vi "总磷氨氮插入数据.vi"(0 "table":string, 1 "关键参数":T1, 5 "data":T3={"时间标识"=timestamp(0 s since 1904-01-01), "测量模式"=enum."水样测试", "数据标记表"="N", "监测值"=0.0, "单位"=0, "数据标识"="", "因子编码"=0, "标样参考值"=0.0, "F0"=0.0, "F1"=0.0, "F2"=0.0, "F3"=0.0, "F4"=0.0, "F5"=0.0, "F6"=0.0, "F7"=0.0, "X"=0.0, "温度"=0.0, "湿度"=0.0, "量程标识"="", "SN"="", "跨度值"=0.0} {"单位" items=["μg/L", "mg/L", "ppm", "mg/m3", "cm", "ppb", "μg/m3", "%", "nmol/mol", "μmol/mol", "MPN/L", "MPN/100ml", "ng/m3", "NTU", "无量纲", "ms/cm", "μs/cm"]}, 11 "error in (no error)":errorcluster) -> (15 "error out":errorcluster)   [LabVIEW 2016, in "斯坦道氨氮.lvlib"]
uses:
  <vilib>/Utility/sysdir.llb/System Directory Type.ctl
  <vilib>/Utility/error.llb/DialogType.ctl
  <vilib>/addons/database/Auxilliary.llb/DB Tools Column Info.ctl
  <vilib>/addons/database/Auxilliary.llb/DB Tools DataTypes.ctl
  <vilib>/addons/database/Connection.llb/DB Tools Open Connec (String).vi
  <vilib>/addons/database/Connection.llb/Conn Execute.vi
  <vilib>/addons/database/Recordset.llb/Rec Fetch Recordset Data (R).vi
  <vilib>/addons/database/Recordset.llb/Rec Destroy - Connection.vi
  <vilib>/addons/database/NI_Database_API.lvlib
  <vilib>/Utility/VariantDataType/VariantType.lvlib
panel:
  out "data输出":T2
  out "为空？":bool
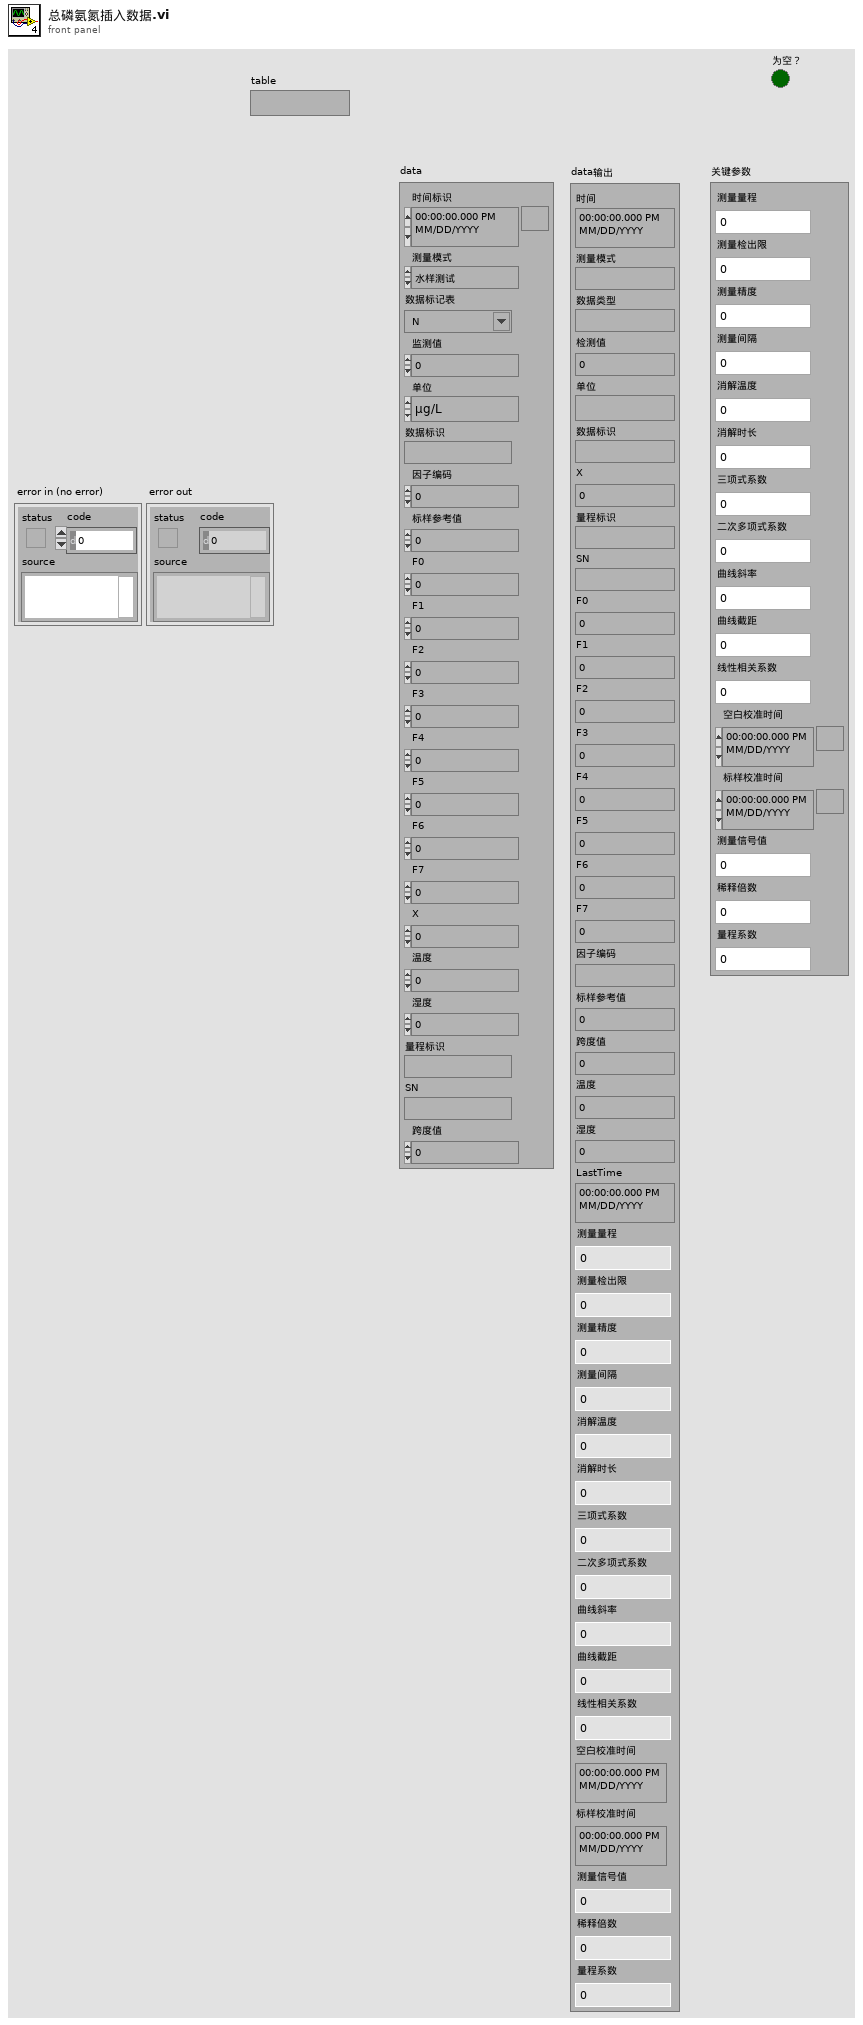
[diagram p1: front panel]
types:
  T1 = typedef "斯坦道氨氮.lvlib/关键参数.ctl" = cluster{"测量量程":sgl, "测量检出限":sgl, "测量精度":sgl, "测量间隔":sgl, "消解温度":sgl, "消解时长":sgl, "三项式系数":sgl, "二次多项式系数":sgl, "曲线斜率":sgl, "曲线截距":sgl, "线性相关系数":sgl, "空白校准时间":timestamp, "标样校准时间":timestamp, "测量信号值":sgl, "稀释倍数":sgl, "量程系数":sgl}
  T2 = cluster{"时间":timestamp, "测量模式":string, "数据类型":string, "检测值":sgl, "单位":string, "数据标识":string, "X":sgl, "量程标识":string, "SN":string, "F0":sgl, "F1":sgl, "F2":sgl, "F3":sgl, "F4":sgl, "F5":sgl, "F6":sgl, "F7":sgl, "因子编码":string, "标样参考值":sgl, "跨度值":sgl, "温度":sgl, "湿度":sgl, "LastTime":timestamp, "测量量程":sgl, "测量检出限":sgl, "测量精度":sgl, "测量间隔":sgl, "消解温度":sgl, "消解时长":sgl, "三项式系数":sgl, "二次多项式系数":sgl, "曲线斜率":sgl, "曲线截距":sgl, "线性相关系数":sgl, "空白校准时间":timestamp, "标样校准时间":timestamp, "测量信号值":sgl, "稀释倍数":sgl, "量程系数":sgl}
  T3 = cluster{"时间标识":timestamp, "测量模式":enum16{"维护数据", "水样测试", "标样核查", "零点核查", "跨度核查", "空白测试", "平行样测试", "加标回收", "空白校准", "标样校准", "初始化（清洗）"}, "数据标记表":string, "监测值":sgl, "单位":u16, "数据标识":string, "因子编码":u32, "标样参考值":sgl, "F0":sgl, "F1":sgl, "F2":sgl, "F3":sgl, "F4":sgl, "F5":sgl, "F6":sgl, "F7":sgl, "X":sgl, "温度":sgl, "湿度":sgl, "量程标识":string, "SN":string, "跨度值":sgl}
  T4 = typedef "DialogType.ctl" = u16
  T5 = typedef "System Directory Type.ctl" = i32
  T6 = typedef "NI_Database_API.lvlib/Conn ObjectReference.ctl" = refnum<k1>
  T7 = typedef "NI_Database_API.lvlib/Rec ObjectReference.ctl" = refnum<k1>
  T8 = typedef "NI_Database_API.lvlib/DB Tools Column Info.ctl" = cluster{"column name":string, "data type":T9, "size":i32, "allow null?":bool}
  T9 = typedef "NI_Database_API.lvlib/DB Tools DataTypes.ctl" = enum16{"String", "Long (I32)", "Single (SGL)", "Double (DBL)", "Date/Time", "Binary"}
  T10 = enum16{"维护数据", "水样测试", "标样核查", "零点核查", "跨度核查", "空白测试", "平行样测试", "加标回收", "空白校准", "标样校准", "初始化（清洗）"}
  T11 = cluster{"测量量程":dbl, "测量精度":dbl, "测量间隔":dbl, "消解温度":dbl, "消解时长":dbl, "空白校准时间":timestamp, "曲线截距":dbl, "曲线斜率":dbl, "测量检出限":dbl, "测量信号值":dbl, "线性相关系数":dbl, "二次多项式系数":dbl, "标样校准时间":timestamp, "稀释倍数":dbl, "三项式系数":dbl, "空白标定系数":dbl, "量程系数":dbl, "F0/ORPA":dbl, "F1/ORPB":dbl, "F2/ORPK":dbl, "F3":dbl, "F4":dbl, "F5":dbl, "F6":dbl, "F7":dbl, "X0/滴定数":dbl, "量程":dbl}
  T12 = typedef "VariantType.lvlib/Type.ctl" = enum8{"Invalid Type", "Void", "I8", "I16", "I32", "I64", "U8", "U16", "U32", "U64", "Single Float", "Double Float", "Extended Float", "Single Complex", "Double Complex", "Extended Complex", "Enum U8", "Enum U16", "Enum U32", "Enum U64", "Single Float With Unit", "Double Float With Unit", "Extended Float With Unit", "Single Complex with Unit", "Double Complex with Unit", "Extended Complex with Unit", "Boolean", "String", "Path", "Picture", "Tag", "Array", "Cluster", "Variant", "LV Variant", "Waveform", "Timestamp", "Digital Waveform", "Digital Data", "ExpressData", "Refnum", "External Data", "VI", "Poly VI", "LabVIEW Class Instance", "Fixed Point"}
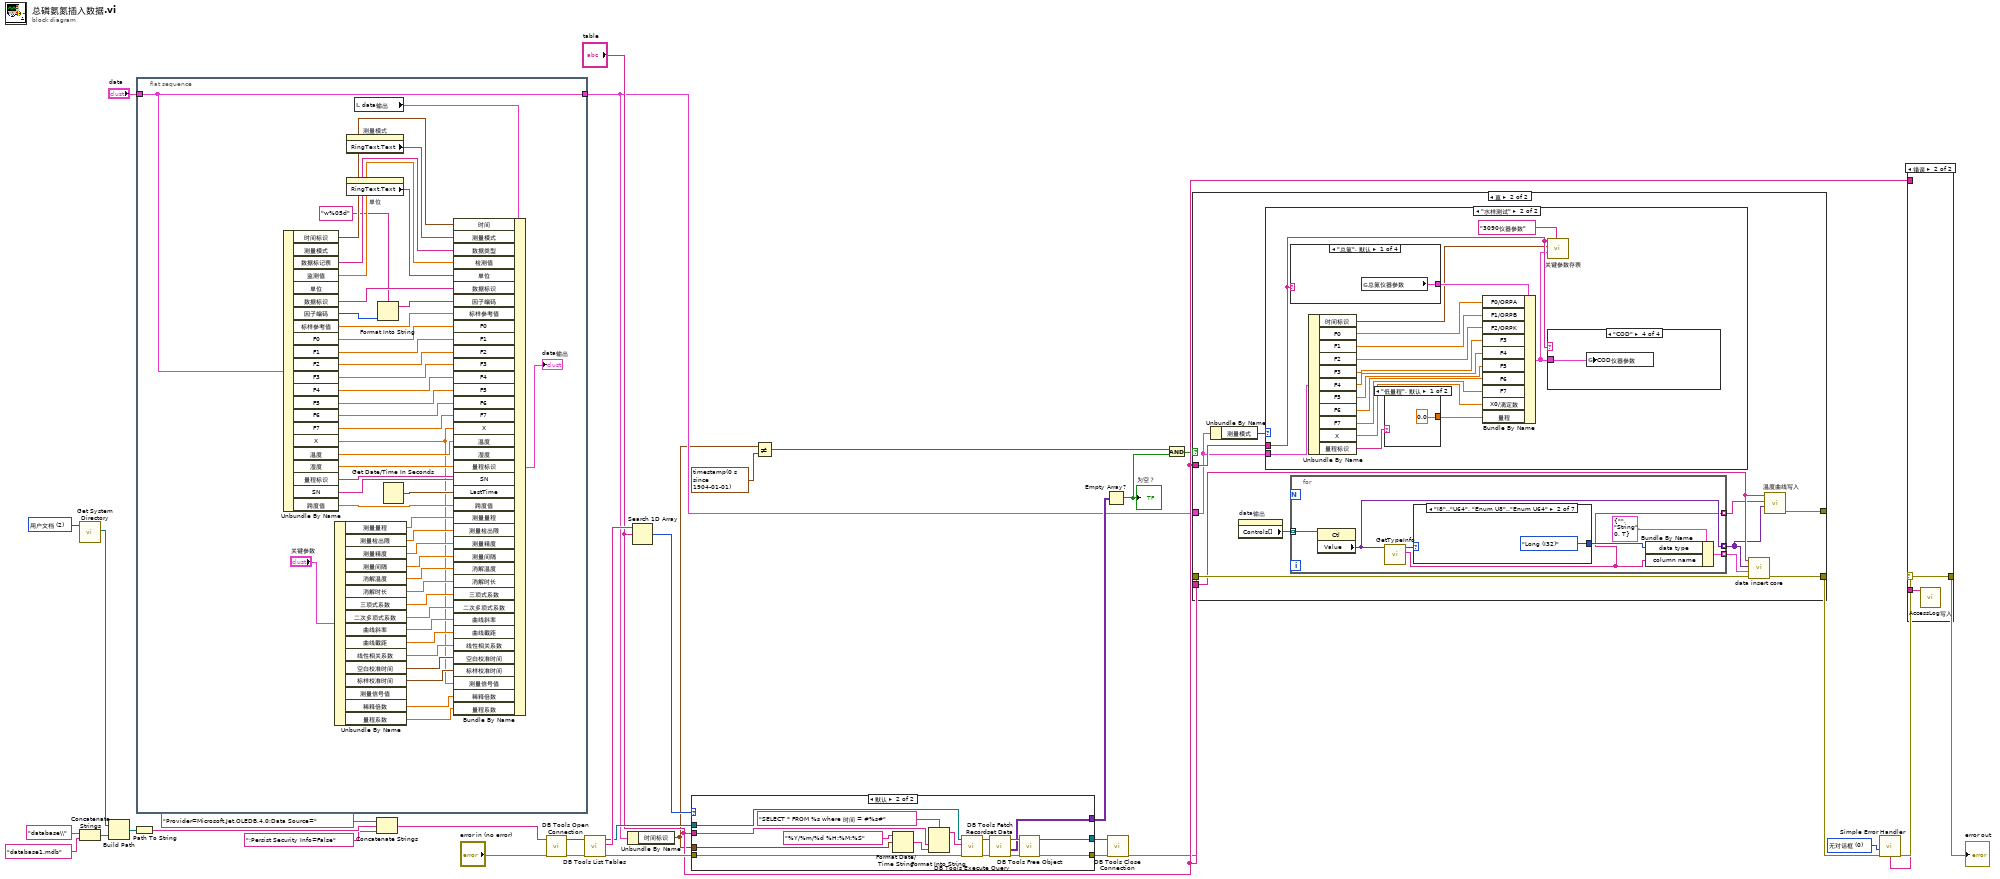
[diagram p0: block diagram]
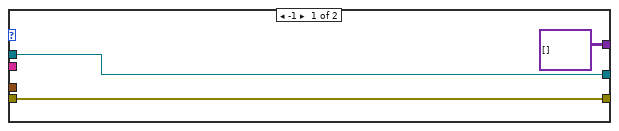
[diagram p3: hidden frame]
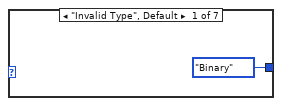
[diagram p5: hidden frame]
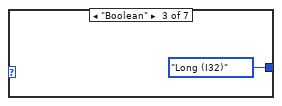
[diagram p6: hidden frame]
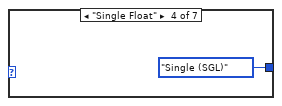
[diagram p7: hidden frame]
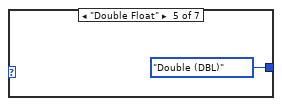
[diagram p8: hidden frame]
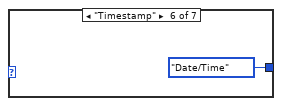
[diagram p9: hidden frame]
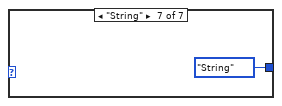
[diagram p10: hidden frame]
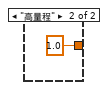
[diagram p12: hidden frame]
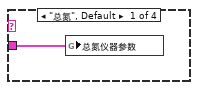
[diagram p13: hidden frame]
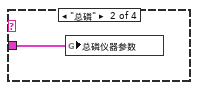
[diagram p14: hidden frame]
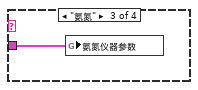
[diagram p15: hidden frame]
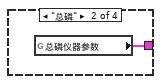
[diagram p16: hidden frame]
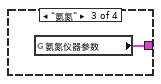
[diagram p17: hidden frame]
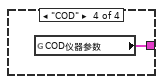
[diagram p18: hidden frame]
diagram:
  w15 = T4 0 items=["无对话框", "确定信息", "继续或停止信息", "确定信息＋警告", "继续/停止+警告"] ("type of dialog (OK msg:1)")
  w33 = T5 2 items=["用户目录"=0, "用户桌面"=1, "用户文档"=2, "用户应用程序数据"=3, "用户设置"=4, "用户临时目录"=5, "公共文档"=6, "公共应用程序数据"=7, "公共设置"=8, "公共缓存"=13, "系统核心库"=9, "系统安装库"=10, "应用程序文件"=11, "启动盘根目录"=12] ("system directory type")
  n1 = call <vilib>:"Get System Directory.vi"("system directory type"=w33) -> ("system directory"=w31:path)  [unwired: 10 in]
  n2 = Concatenate Strings("database\\" ("condition"), "database1.mdb" ("database")) -> (w25:string)
  n3 = Build Path(base path=w31, name or relative path=w25) -> (appended path=w30:path)
  n4 = Path To String(path=w30) -> (string=w29:string)
  n5 = flat-sequence {
    tunnel: "data" -> [w57]
    tunnel: [w57] -> w9
    frame #0 {
      n6 = Unbundle By Name(w57) -> ("时间标识"=w77:timestamp, "数据标记表"=w75:string, "监测值"=w74:sgl, "数据标识"=w72:string, "因子编码"=w56:u32, "标样参考值"=w71:sgl, "F0"=w70:sgl, "F1"=w69:sgl, "F2"=w68:sgl, "F3"=w67:sgl, "F4"=w66:sgl, "F5"=w65:sgl, "F6"=w64:sgl, "F7"=w63:sgl, "X"=w35:sgl, "温度"=w62:sgl, "湿度"=w61:sgl, "量程标识"=w60:string, "SN"=w59:string, "跨度值"=w52:sgl)  [unwired: 2 out]
      n7 = Unbundle By Name("关键参数") -> ("测量量程"=w50:sgl, "测量检出限"=w49:sgl, "测量精度"=w48:sgl, "测量间隔"=w47:sgl, "消解温度"=w46:sgl, "消解时长"=w45:sgl, "三项式系数"=w44:sgl, "二次多项式系数"=w43:sgl, "曲线斜率"=w42:sgl, "曲线截距"=w41:sgl, "线性相关系数"=w40:sgl, "空白校准时间"=w39:timestamp, "标样校准时间"=w38:timestamp, "稀释倍数"=w37:sgl, "量程系数"=w36:sgl)  [unwired: 1 out]
      n8 = property on="测量模式" class="Enum (严格)"() -> ("RingText.Text"=w76:string)  [unwired: 2 in, 2 out]
      n9 = property on="单位" class="Ring (严格)"() -> ("RingText.Text"=w73:string)  [unwired: 2 in, 2 out]
      n10 = local read "data输出"() -> (w53:T2)
      n11 = Format Into String(format string="w%05d" ("格式字符串"), w56) -> (resulting string=w54:string)  [unwired: 2 in, 1 out]
      n12 = Get Date/Time In Seconds() -> (seconds since 1Jan1904=w58:timestamp)
      n13 = Bundle By Name(cluster=w53, "时间"=w77, "测量模式"=w76, "数据类型"=w75, "检测值"=w74, "单位"=w73, "数据标识"=w72, "因子编码"=w54, "标样参考值"=w71, "F0"=w70, "F1"=w69, "F2"=w68, "F3"=w67, "F4"=w66, "F5"=w65, "F6"=w64, "F7"=w63, "X"=w35, "温度"=w62, "湿度"=w61, "量程标识"=w60, "SN"=w59, "LastTime"=w58, "跨度值"=w52, "测量量程"=w50, "测量检出限"=w49, "测量精度"=w48, "测量间隔"=w47, "消解温度"=w46, "消解时长"=w45, "三项式系数"=w44, "二次多项式系数"=w43, "曲线斜率"=w42, "曲线截距"=w41, "线性相关系数"=w40, "空白校准时间"=w39, "标样校准时间"=w38, "测量信号值"=w35, "稀释倍数"=w37, "量程系数"=w36) -> (→"data输出":T2)
    }
  }
  n14 = Concatenate Strings("Provider=Microsoft.Jet.OLEDB.4.0;Data Source=" ("condition"), w29, ";Persist Security Info=False" ("condition")) -> (w27:string)
  n15 = call-poly <vilib>:"DB Tools Open Connection.vi"("error in (no error)"="error in (no error)", "connection information"=w27) -> ("error out"=w23:errorcluster, "connection reference"=w24:T6)  [unwired: 6 in]
  n16 = call <vilib>:"DB Tools List Tables.vi"("error in (no error)"=w23, "connection reference"=w24) -> ("error out"=w17:errorcluster, "tables"=w22:string[], "connection reference out"=w18:T6)  [unwired: 3 in]
  n17 = Unbundle By Name(w9) -> ("时间标识"=w7:timestamp)
  n18 = Search 1D Array(1D array=w22, element="table") -> (index of element=w19:i32)  [unwired: 1 in]
  n19 = case shown="默认" w19 {
    tunnel: [variant[][] [] ("recordset data") w92] -> w16
    tunnel: [w81 w83] -> w4
    tunnel: [w80 w91] -> w3
    tunnel: w18 -> [w81 w87]
    tunnel: w17 -> [w80 w86]
    tunnel: "table" -> [_ w85]
    tunnel: w7 -> [_ w82]
    frame -1 {
    }
    frame Default {
      n20 = Format Date/Time String(time format string (%c)="%Y/%m/%d %H:%M:%S" ("时间格式字符串(%c)"), seconds (now)=w82) -> (date/time string=w88:string)  [unwired: 1 in]
      n21 = Format Into String(format string="SELECT * FROM %s where 时间 = #%s#" ("格式字符串"), w85, w88) -> (resulting string=w90:string)  [unwired: 2 in, 1 out]
      n22 = call-poly <vilib>:"DB Tools Execute Query.vi"("error in (no error)"=w86, "SQL query"=w90, "connection reference"=w87) -> ("error out"=w93:errorcluster, "recordset reference"=w96:T7)  [unwired: 5 in]
      n23 = call-poly <vilib>:"DB Tools Fetch Recordset Data.vi"("error in (no error)"=w93, "recordset reference"=w96) -> ("error out"=w94:errorcluster, "recordset data"=w92:variant[][], "recordset reference out"=w95:T7)  [unwired: 3 in]
      n24 = call-poly <vilib>:"DB Tools Free Object.vi"("error in (no error)"=w94, "recordset reference"=w95) -> ("error out"=w91:errorcluster, "connection reference"=w83:T6)  [unwired: 8 in]
    }
  }
  n25 = Not Equal?(x=w7, y=timestamp(0 s since 1904-01-01)) -> (x != y?=w5:bool)
  n26 = Empty Array?(array=w16) -> (empty?=w20:bool)
  "为空？" <- w20
  n27 = call <vilib>:"DB Tools Close Connection.vi"("error in (no error)"=w3, "connection reference"=w4) -> ("error out"=w2:errorcluster)  [unwired: 5 in]
  n28 = And(x=w5, y=w20) -> (x .and. y?=w6:bool)
  n29 = case shown="真" w6 {
    tunnel: "table" -> [_ w101]
    tunnel: w9 -> [_ w106]
    tunnel: w2 -> [w97 w102]
    tunnel: [w97 w107] -> w1
    tunnel: "table" -> [_ w108]
    tunnel: [_ w100] -> _
    frame False {
    }
    frame True {
      n30 = Unbundle By Name(w106) -> ("测量模式"=w105:T10)
      n31 = property on="data输出" class="Clust (严格)"() -> ("Controls[]"=w104:refnum<vi>[])  [unwired: 2 in, 2 out]
      n32 = case shown="\"水样测试\"" w105 {
        tunnel: w106 -> [_ w138]
        tunnel: w108 -> [_ w136]
        frame "维护数据", Default {
        }
        frame "水样测试" {
          n33 = case shown="\"总氮\", 默认" w136 {
            tunnel: [w146 w147 w148 w149] -> w137
            frame "总氮", Default {
              n34 = global read "总磷总氮断电保存全局变量.vi" "总氮仪器参数"() -> (w146:T11)
            }
            frame "总磷" {
              n35 = global read "总磷总氮断电保存全局变量.vi" "总磷仪器参数"() -> (w147:T11)
            }
            frame "氨氮" {
              n36 = global read "总磷总氮断电保存全局变量.vi" "氨氮仪器参数"() -> (w148:T11)
            }
            frame "COD" {
              n37 = global read "总磷总氮断电保存全局变量.vi" "COD仪器参数"() -> (w149:T11)
            }
          }
          n38 = Unbundle By Name(w138) -> ("时间标识"=w134:timestamp, "F0"=w123:sgl, "F1"=w124:sgl, "F2"=w125:sgl, "F3"=w126:sgl, "F4"=w127:sgl, "F5"=w128:sgl, "F6"=w129:sgl, "F7"=w130:sgl, "X"=w131:sgl, "量程标识"=w133:string)
          n39 = case shown="\"低量程\", 默认" w133 {
            tunnel: [0.0 1.0] -> w132
            frame "低量程", Default {
            }
            frame "高量程" {
            }
          }
          n40 = Bundle By Name(cluster=w137, "F0/ORPA"=w123, "F1/ORPB"=w124, "F2/ORPK"=w125, "F3"=w126, "F4"=w127, "F5"=w128, "F6"=w129, "F7"=w130, "X0/滴定数"=w131, "量程"=w132) -> (w135:T11)
          n41 = call "关键参数存表.vi"("table"="3090仪器参数", "仪器参数"=w135, "datatime"=w134, "仪器名称"=w136) -> ()  [unwired: 7 in, 1 out]
          n42 = case shown="\"COD\"" w136 {
            tunnel: w135 -> [w142 w143 w144 w145]
            frame "总氮", Default {
              n43 = global write "总磷总氮断电保存全局变量.vi" "总氮仪器参数"(w142) -> ()
            }
            frame "总磷" {
              n44 = global write "总磷总氮断电保存全局变量.vi" "总磷仪器参数"(w143) -> ()
            }
            frame "氨氮" {
              n45 = global write "总磷总氮断电保存全局变量.vi" "氨氮仪器参数"(w144) -> ()
            }
            frame "COD" {
              n46 = global write "总磷总氮断电保存全局变量.vi" "COD仪器参数"(w145) -> ()
            }
          }
        }
      }
      n47 = for {
        tunnel: w104 -> [w115] mode=indexing
        tunnel: [w110] -> w98 mode=indexing
        tunnel: [w111] -> w103 mode=indexing
        tunnel: [w109] -> w99 mode=indexing
        n48 = property class="Ctl"(reference=w115) -> ("Value"=w110:variant)  [unwired: 1 in, 2 out]
        n49 = call <vilib>:"GetTypeInfo.vi"("Variant"=w110) -> ("Name"=w109:string, "Type Enum"=w113:T12)  [unwired: 6 in, 3 out]
        n50 = case shown="\"I8\"..\"U64\", \"Enum U8\"..\"Enum U64\"" w113 {
          tunnel: [DB_Tools_DataTypes."Binary" ("data type") DB_Tools_DataTypes."Long (I32)" ("data type") DB_Tools_DataTypes."Long (I32)" ("data type") DB_Tools_DataTypes."Single (SGL)" ("data type") DB_Tools_DataTypes."Double (DBL)" ("data type") DB_Tools_DataTypes."Date/Time" ("data type") DB_Tools_DataTypes."String" ("data type")] -> w112
          frame "Invalid Type", Default {
          }
          frame "I8".."U64", "Enum U8".."Enum U64" {
          }
          frame "Boolean" {
          }
          frame "Single Float" {
          }
          frame "Double Float" {
          }
          frame "Timestamp" {
          }
          frame "String" {
          }
        }
        n51 = Bundle By Name(cluster=T8 {"column name"="", "data type"=enum."String", "size"=0, "allow null?"=TRUE} ("column information"), "data type"=w112, "column name"=w109) -> (w111:T8)
      }
      n52 = call "data insert core.vi"("error in (no error)"=w102, "column information"=w103, "data"=w98, "table"=w101) -> ("error out"=w107:errorcluster)  [unwired: 7 in]
      n53 = call "温度曲线写入.vi"("属性值"=w98, "属性名称"=w99, "table"=w101) -> ("错误输出"=w100:errorcluster)  [unwired: 8 in]
    }
  }
  n54 = call <vilib>:"Simple Error Handler.vi"("type of dialog (OK msg:1)"=w15, "error in (no error)"=w1) -> ("error out"=w14:errorcluster, "message"=w13:string)  [unwired: 3 in, 3 out]
  n55 = case shown="错误" w14 {
    selector: w14 -> [_ w150]
    tunnel: w13 -> [_ w151]
    tunnel: [_ w150] -> w12
    tunnel: "table" -> [_ _]
    frame No Error {
    }
    frame Error {
      n56 = call "AccessLog写入.vi"("Log"=w151) -> ()  [unwired: 11 in]
    }
  }
  "error out" <- w12
